vi "Calibration curve generator, inverse (for plot visualisation).vi"(0 "Calibration data":T1={"X cal.[]"=[0.18323830295620053, 0.5022759108677167, 0.5926494582411277, 0.6661572393359195, 0.7738522670991032, 0.8056162976693839, 0.8978854253288069, 0.9131465104685323, 0.998198602505461, 1.0026536354542668, 1.0697031684682123, 1.0921294784978217, 1.12634848007751], "Re cal.[]"=[0.05836901900647489, 0.22234941748039563, 0.3015014894413766, 0.37907259878050203, 0.5315212662031547, 0.5843186336351215, 0.7493379557739939, 0.7811312845686427, 0.9579100635301298, 0.968544779466997, 1.1278235480081842, 1.1845542549316277, 1.2707750850078616], "a1[]"=[0.5139845410306613, 0.694908421100499, 0.9655549133380104, 1.2354182702612118, 1.5388668488196042, 1.7253155968767342, 1.935875310920986, 2.080885331144939, 2.2328002605238204, 2.3813313947618693, 2.452594226248764, 2.5246632991683033], "a2[]"=[-0.567092642319511, 3.0111150428522957, -0.009461861177446703, 2.2004140825264833, 5.776179850523374, -0.22907956125341525, 19.477407826803766, -1.871103511573675, 70.58084557623488, -1.3220160025433672, 7.094218596447346, -0.2914365144530001], "a3[]"=[1.7775103256064757, -11.166529475918521, 16.733581628717324, -4.900141213800908, -59.63298736273686, 9.899216022714324, -643.3109334585097, 21.66651332028892, -8067.401298929666, 18.428518110921583, -163.1245085960374, 4.25840177969994]}, 5 "Overheat ratio":dbl=1.7, 7 "Gain":dbl=10.0, 9 "Offset (V)":dbl=0.512, 11 "N pts":i32=200, 12 "U_start (m/s)":dbl=0.3, 13 "U_end (m/s)":dbl=6.45, 14 "Ta (°C)":dbl=20.4383) -> ()   [LabVIEW 2022 SP3]
doc: "Generate spline interpolated calibration curve for plotting or testing purposes, inverse.\nPN 15-OCT-24."
uses:
  Ctls/Calibration data.ctl
  <vilib>/Analysis/1siggen.llb/Ramp Pattern by Samples.vi
  <vilib>/Analysis/NI_AALBase.lvlib
panel:
  out "U against Vout":cluster{dbl[], dbl[]}(graph)={[0.09565670008978011, 0.1343898964717316, 0.1737745519320799, 0.21373098990741246, 0.25415906989051273, 0.29493850771461716, 0.33593072128072055, 0.37698235326171226, 0.4179303781005761, 0.4586084143648783, 0.4988536102025265, 0.5385133294924527, 0.5774508898457986, 0.6155497865817461, 0.6527161209334209, 0.6888792508070907, 0.7239909224791807, 0.7580232803409792, 0.7909661871209617, 0.8228242441965239, 0.8536138157916306, 0.8833602633133519, 0.9120955076928228, 0.9398559684447683, 0.9666808802820959, 0.992610958957687, 1.017687373168673, 1.0419404638648222, 1.0648307784179123, 1.0863400234648268, 1.1067816169742883, 1.1263773140464783, 1.1452918887230468, 1.1636527433939259, 1.1815617818976187, 1.199103010231084, 1.216347641088802, 1.2333576762724352, 1.250188532885781, 1.2668910603604677, 1.2835131302849823, 1.3000737074622026, 1.3165183307523298, 1.3327837302632117, 1.3488125367586157, 1.3645549977294102, 1.3799700065077525, 1.3950254497808412, 1.409697968131386, 1.423972276022466, 1.4378402016851988, 1.4512995928993822, 1.4643532042626861, 1.4770174447515505, 1.489413910082965, 1.501590738566163, 1.5135643030588108, 1.5253492940795044, 1.5369589601284572, 1.5484053060396363, 1.5596992580108715, 1.5708508019310274, 1.5818691001255758, 1.592762590522131, 1.6035390713912545, 1.6142057741717097, 1.6247694263914259, 1.6352363063082798, 1.6456122905913884, 1.6559028961239342, 1.666113316817932, 1.6762484561786817, 1.6863129562336754, 1.6963112233410027, 1.706247451311157, 1.7161256422095328, 1.7259496251522843, 1.7357230733629458, 1.7454390277558163, 1.7549380938176284, 1.7642040931670222, 1.773280174660391, 1.782202692841075, 1.7910030846456615, 1.7997092295949835, 1.8083464784953251, 1.8169384687602363, 1.8255089240700306, 1.8340734713718665, 1.8426296175162848, 1.851173732752187, 1.8597022115890582, 1.8682114881290202, 1.8766980510068698, 1.8851584577645808, 1.893589348498953, 1.9019874586367636, 1.9103496307103862, 1.918672825027632, 1.9269541291519754, 1.9351907661324885, 1.943380101446166, 1.9515196486379371, 1.9596070736653148, 1.967640197974384, 1.9756170003516893, 1.9835356176118912, 1.9913943441939108, 1.9991916307484203, 2.00692608180709, 2.0145964526289784, 2.022201645322114, 2.029740704338787, 2.037212811441754, 2.044577031371202, 2.051621627394792, 2.0584422040883785, 2.0651575965089783, 2.071870086802438, 2.0786774895385776, 2.085550101994925, 2.092448142234443, 2.0993681711684484, 2.10630661311665, 2.1132597718178756, 2.1202238482677527, 2.127194960174401, 2.134169162776134, 2.141142470723861, 2.1481108806974722, 2.155070394401509, 2.162017041572377, 2.1689469026275665, 2.175856130597331, 2.18274097200035, 2.189597786355985, 2.1964230640655034, 2.2032134424409824, 2.2099657197115032, 2.216676866889371, 2.223344037432353, 2.229964574689168, 2.23653601716303, 2.243056101670474, 2.2495227645090354, 2.255934140776863, 2.2622885620099376, 2.2685845523181625, 2.274808698274382, 2.2806124757935544, 2.2863813895656646, 2.2922116126597114, 2.2980513875361175, 2.3038989912036323, 2.309752668696791, 2.3156106380566333, 2.32147109555613, 2.3273322211294523, 2.333192183960767, 2.3390491481853672, 2.344901278653928, 2.350746746709451, 2.3565837359260398, 2.3624104477592334, 2.3682251070589535, 2.374025967398322, 2.3798113161745906, 2.3855794794420593, 2.3913288264411303, 2.3970577737923513, 2.402764789329379, 2.408448395550149, 2.414107172670926, 2.4197397612733518, 2.4253448645398867, 2.430921250078122, 2.436466557075516, 2.44194958964132, 2.447368419589284, 2.45273726628724, 2.458069198680594, 2.463376486348948, 2.4686708978236394, 2.473963967621354, 2.479267249448951, 2.4845925713516106, 2.4899364329103912, 2.4952794764099337, 2.5006211554658653, 2.50596116144255, 2.511299185353878, 2.516634918044822, 2.521968050373835, 2.5272982733957337, 2.532625278544789, 2.537948757817723, 2.543268403956315, 2.5485839106292785, 2.5538949726131643, 2.559201285971937], [0.3, 0.3309045226130653, 0.36180904522613067, 0.392713567839196, 0.4236180904522613, 0.4545226130653266, 0.48542713567839196, 0.5163316582914572, 0.5472361809045226, 0.578140703517588, 0.6090452261306533, 0.6399497487437186, 0.670854271356784, 0.7017587939698493, 0.7326633165829146, 0.7635678391959799, 0.7944723618090452, 0.8253768844221105, 0.8562814070351759, 0.8871859296482412, 0.9180904522613065, 0.9489949748743718, 0.9798994974874371, 1.0108040201005026, 1.041708542713568, 1.0726130653266333, 1.1035175879396986, 1.1344221105527639, 1.1653266331658292, 1.1962311557788945, 1.2271356783919598, 1.2580402010050251, 1.2889447236180904, 1.319849246231156, 1.3507537688442213, 1.3816582914572866, 1.412562814070352, 1.4434673366834172, 1.4743718592964825, 1.5052763819095478, 1.5361809045226131, 1.5670854271356784, 1.5979899497487438, 1.628894472361809, 1.6597989949748744, 1.69070351758794, 1.7216080402010052, 1.7525125628140705, 1.7834170854271358, 1.8143216080402012, 1.8452261306532665, 1.8761306532663318, 1.907035175879397, 1.9379396984924624, 1.9688442211055277, 1.999748743718593, 2.030653266331658, 2.0615577889447234, 2.092462311557789, 2.1233668341708545, 2.15427135678392, 2.185175879396985, 2.2160804020100504, 2.2469849246231157, 2.277889447236181, 2.3087939698492463, 2.3396984924623117, 2.370603015075377, 2.4015075376884423, 2.4324120603015076, 2.463316582914573, 2.494221105527638, 2.5251256281407035, 2.556030150753769, 2.586934673366834, 2.6178391959798994, 2.6487437185929648, 2.67964824120603, 2.7105527638190954, 2.7414572864321607, 2.772361809045226, 2.8032663316582913, 2.8341708542713566, 2.865075376884422, 2.8959798994974872, 2.9268844221105526, 2.957788944723618, 2.988693467336683, 3.0195979899497485, 3.050502512562814, 3.0814070351758795, 3.112311557788945, 3.14321608040201, 3.1741206030150755, 3.205025125628141, 3.235929648241206, 3.2668341708542714, 3.2977386934673367, 3.328643216080402, 3.3595477386934673, 3.3904522613065327, 3.421356783919598, 3.4522613065326633, 3.4831658291457286, 3.514070351758794, 3.544974874371859, 3.5758793969849245, 3.60678391959799, 3.637688442211055, 3.6685929648241205, 3.6994974874371858, 3.730402010050251, 3.7613065326633164, 3.7922110552763817, 3.823115577889447, 3.8540201005025123, 3.884924623115578, 3.9158291457286434, 3.9467336683417087, 3.977638190954774, 4.00854271356784, 4.039447236180905, 4.07035175879397, 4.101256281407036, 4.132160804020101, 4.163065326633166, 4.193969849246232, 4.224874371859297, 4.255778894472362, 4.2866834170854275, 4.317587939698493, 4.348492462311558, 4.3793969849246235, 4.410301507537689, 4.441206030150754, 4.472110552763819, 4.503015075376885, 4.53391959798995, 4.564824120603015, 4.595728643216081, 4.626633165829146, 4.657537688442211, 4.688442211055277, 4.719346733668342, 4.750251256281407, 4.7811557788944725, 4.812060301507538, 4.842964824120603, 4.8738693467336685, 4.904773869346734, 4.935678391959799, 4.966582914572864, 4.99748743718593, 5.028391959798995, 5.05929648241206, 5.090201005025126, 5.121105527638191, 5.152010050251256, 5.182914572864322, 5.213819095477387, 5.244723618090452, 5.2756281407035175, 5.306532663316583, 5.337437185929648, 5.368341708542713, 5.399246231155779, 5.430150753768844, 5.461055276381909, 5.491959798994975, 5.52286432160804, 5.553768844221105, 5.584673366834171, 5.615577889447236, 5.646482412060301, 5.6773869346733665, 5.708291457286432, 5.739195979899497, 5.7701005025125625, 5.801005025125628, 5.831909547738693, 5.862814070351759, 5.893718592964825, 5.92462311557789, 5.955527638190955, 5.9864321608040205, 6.017336683417086, 6.048241206030151, 6.0791457286432165, 6.110050251256282, 6.140954773869347, 6.171859296482412, 6.202763819095478, 6.233668341708543, 6.264572864321608, 6.295477386934674, 6.326381909547739, 6.357286432160804, 6.38819095477387, 6.419095477386935, 6.45]}
  out "Calibration curve":cluster{dbl[], dbl[]}(graph)={[0.18451097716861914, 0.19652537347054594, 0.20883298963589056, 0.22141320587161856, 0.23423819544835056, 0.2472727548728119, 0.26047463068740484, 0.27379542336054125, 0.28718207192142786, 0.3005788254708218, 0.31392951339678693, 0.32717986335272775, 0.3402796056958915, 0.3531841487174906, 0.365855695129608, 0.3782637698457373, 0.3903852154178121, 0.40220376777841, 0.41370934729013237, 0.4248971946349325, 0.4357669584395782, 0.44632181214277844, 0.45656764901945185, 0.46651238062858197, 0.476165346624981, 0.48553683253197344, 0.4946376855652234, 0.5034751781541572, 0.5118480638703804, 0.5197440706361511, 0.5272735497260558, 0.5345146935617827, 0.5415257237079875, 0.5483517836440789, 0.5550291144751378, 0.5615877309369915, 0.5680532220324355, 0.574448018846105, 0.5807923288016678, 0.5871048588876737, 0.5934033913908016, 0.5996949027790756, 0.6059584418879481, 0.6121694791887384, 0.6183055074963921, 0.6243467367193586, 0.6302765339708374, 0.6360816054103551, 0.6417519511197015, 0.647280645556046, 0.6526635030850395, 0.6578986839495075, 0.6629862854029505, 0.667931779891953, 0.6727819095589543, 0.6775549708575999, 0.6822569237172977, 0.6868931198680651, 0.6914683899511406, 0.6959871154220011, 0.7004532883800795, 0.7048705617244951, 0.7092422914921751, 0.7135715728288287, 0.717861270736505, 0.722114046507269, 0.7263323805720736, 0.7305185923535991, 0.7346748576018877, 0.7388032236047495, 0.7429056225958743, 0.7469838836282733, 0.7510397431361439, 0.7550748543721464, 0.7590907958777113, 0.7630890791199043, 0.7670711554086191, 0.7710384221915293, 0.7749879608006575, 0.7788547416735615, 0.7826317994234272, 0.7863363737405534, 0.7899830259774788, 0.7935843855958696, 0.7971516922374349, 0.8006952069303505, 0.8042245394401007, 0.8077493836919192, 0.8112761457970955, 0.8148037882201684, 0.8183307989034609, 0.8218556684935193, 0.8253768967804789, 0.8288929990284882, 0.8324025121231073, 0.8359040004658274, 0.8393960615516053, 0.8428773311723734, 0.8463464881975853, 0.8498022588917484, 0.8532434207382498, 0.8566688057483318, 0.86007730324347, 0.8634678621085019, 0.8668394925212949, 0.8701912671724579, 0.8735223219953733, 0.8768318564325941, 0.8801191332693794, 0.8833834780687708, 0.8866242782452292, 0.8898409818154629, 0.8930330958657748, 0.8962001847751999, 0.8993247820360901, 0.9023167718094229, 0.9052164174744409, 0.9080740389004627, 0.9109330956825705, 0.9138353052238143, 0.9167681010577989, 0.9197145620290823, 0.922673248214591, 0.92564265566199, 0.9286212229289171, 0.9316073384512384, 0.9345993486571023, 0.937595566722432, 0.9405942818447109, 0.9435937688962538, 0.946592298306478, 0.9495881460155551, 0.9525796033395557, 0.9555649865899938, 0.9585426462983452, 0.9615109759082291, 0.9644684198139852, 0.9674134806434742, 0.9703447257042379, 0.9732607925346676, 0.9761603935246739, 0.9790423195925368, 0.9819054429254521, 0.9847487188100789, 0.987571186595719, 0.9903719698462261, 0.993150275747306, 0.995905393843459, 0.9986313815879183, 1.0011753287660317, 1.003705972126855, 1.0062655134444942, 1.0088312671174489, 1.011402485155225, 1.0139784031162342, 1.0165582422395538, 1.0191412116966452, 1.0217265109457183, 1.0243133321697613, 1.0269008627778182, 1.029488287948065, 1.0320747931904932, 1.0346595669066665, 1.0372418029240857, 1.0398207029831326, 1.0423954791553554, 1.0449653561730352, 1.0475295736514572, 1.050087388187049, 1.052638075316576, 1.0551809313247011, 1.057715274889572, 1.0602404485584174, 1.0627558200475489, 1.0652607833634884, 1.0677547597442336, 1.070236663710926, 1.072692487046901, 1.0751213044997503, 1.0775294344056343, 1.0799226971802045, 1.0823065708871378, 1.0846863238844942, 1.0870671340573013, 1.089454202411306, 1.0918528680992148, 1.0942615736420562, 1.0966716021014082, 1.099082705989238, 1.1014947445528838, 1.1039075764910384, 1.106321060035682, 1.1087350530347946, 1.1111494130356936, 1.1135639973688662, 1.1159786632321642, 1.1183932677752186, 1.1208076681839283, 1.1232217217648968, 1.1256352860296606], [0.059022239021742466, 0.06510241942347976, 0.07118259982521706, 0.07726278022695435, 0.08334296062869162, 0.08942314103042892, 0.09550332143216621, 0.10158350183390348, 0.1076636822356408, 0.11374386263737808, 0.11982404303911538, 0.12590422344085264, 0.13198440384258997, 0.13806458424432724, 0.14414476464606454, 0.15022494504780184, 0.15630512544953912, 0.1623853058512764, 0.1684654862530137, 0.174545666654751, 0.18062584705648826, 0.18670602745822554, 0.19278620785996284, 0.19886638826170014, 0.20494656866343747, 0.21102674906517474, 0.217106929466912, 0.2231871098686493, 0.2292672902703866, 0.23534747067212386, 0.2414276510738612, 0.24750783147559846, 0.2535880118773357, 0.25966819227907306, 0.26574837268081036, 0.27182855308254766, 0.2779087334842849, 0.2839889138860222, 0.2900690942877595, 0.2961492746894968, 0.30222945509123406, 0.30830963549297136, 0.3143898158947086, 0.32046999629644596, 0.32655017669818326, 0.33263035709992056, 0.33871053750165786, 0.3447907179033951, 0.3508708983051324, 0.3569510787068697, 0.36303125910860695, 0.36911143951034425, 0.3751916199120816, 0.3812718003138188, 0.38735198071555615, 0.39343216111729346, 0.3995123415190307, 0.40559252192076795, 0.4116727023225053, 0.4177528827242426, 0.4238330631259799, 0.42991324352771715, 0.43599342392945445, 0.4420736043311918, 0.44815378473292905, 0.45423396513466635, 0.46031414553640365, 0.4663943259381409, 0.4724745063398782, 0.4785546867416155, 0.48463486714335274, 0.49071504754509004, 0.49679522794682734, 0.5028754083485646, 0.5089555887503019, 0.5150357691520392, 0.5211159495537765, 0.5271961299555138, 0.5332763103572511, 0.5393564907589883, 0.5454366711607257, 0.551516851562463, 0.5575970319642002, 0.5636772123659375, 0.5697573927676748, 0.5758375731694121, 0.5819177535711494, 0.5879979339728867, 0.5940781143746239, 0.6001582947763612, 0.6062384751780985, 0.6123186555798359, 0.6183988359815732, 0.6244790163833105, 0.6305591967850478, 0.6366393771867851, 0.6427195575885223, 0.6487997379902596, 0.6548799183919969, 0.6609600987937342, 0.6670402791954715, 0.6731204595972088, 0.679200639998946, 0.6852808204006833, 0.6913610008024206, 0.6974411812041579, 0.7035213616058952, 0.7096015420076325, 0.7156817224093697, 0.721761902811107, 0.7278420832128443, 0.7339222636145816, 0.740002444016319, 0.7460826244180563, 0.7521628048197935, 0.7582429852215308, 0.7643231656232682, 0.7704033460250055, 0.7764835264267427, 0.78256370682848, 0.7886438872302174, 0.7947240676319547, 0.8008042480336919, 0.8068844284354292, 0.8129646088371665, 0.8190447892389038, 0.8251249696406411, 0.8312051500423785, 0.8372853304441156, 0.8433655108458529, 0.8494456912475903, 0.8555258716493276, 0.8616060520510649, 0.8676862324528022, 0.8737664128545394, 0.8798465932562767, 0.885926773658014, 0.8920069540597513, 0.8980871344614886, 0.9041673148632258, 0.9102474952649631, 0.9163276756667004, 0.9224078560684377, 0.928488036470175, 0.9345682168719123, 0.9406483972736495, 0.9467285776753868, 0.9528087580771241, 0.9588889384788614, 0.9649691188805987, 0.971049299282336, 0.9771294796840732, 0.9832096600858105, 0.9892898404875479, 0.9953700208892852, 1.0014502012910225, 1.0075303816927597, 1.0136105620944968, 1.0196907424962343, 1.0257709228979714, 1.0318511032997089, 1.037931283701446, 1.0440114641031835, 1.0500916445049207, 1.0561718249066578, 1.0622520053083953, 1.0683321857101327, 1.0744123661118699, 1.0804925465136073, 1.0865727269153445, 1.0926529073170816, 1.098733087718819, 1.1048132681205562, 1.1108934485222937, 1.1169736289240308, 1.123053809325768, 1.1291339897275054, 1.1352141701292426, 1.14129435053098, 1.1473745309327172, 1.1534547113344549, 1.159534891736192, 1.1656150721379295, 1.1716952525396667, 1.1777754329414039, 1.1838556133431413, 1.1899357937448785, 1.1960159741466159, 1.202096154548353, 1.2081763349500905, 1.2142565153518277, 1.220336695753565, 1.2264168761553023, 1.2324970565570394, 1.2385772369587769, 1.244657417360514, 1.2507375977622515, 1.2568177781639887, 1.2628979585657258, 1.2689781389674633]}
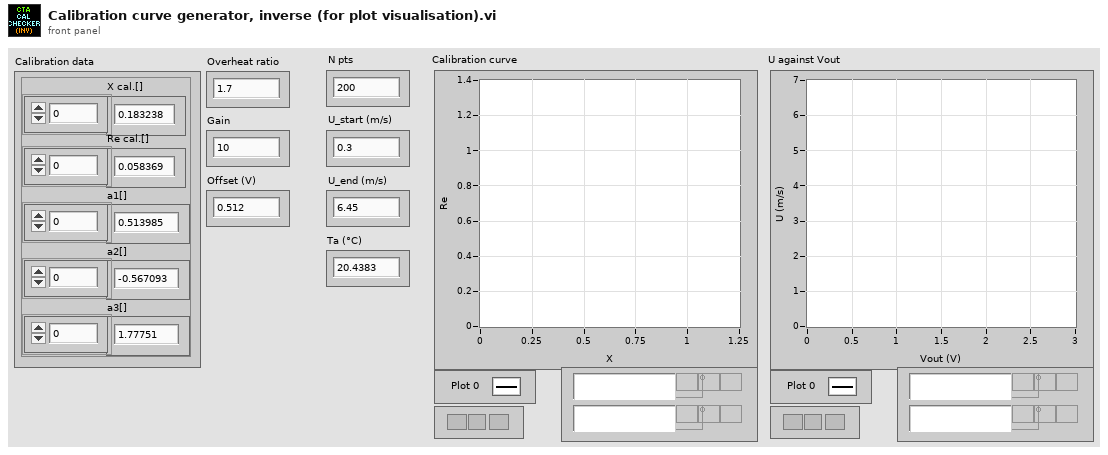
[diagram p1: front panel]
types:
  T1 = typedef "Calibration data.ctl" = cluster{"X cal.[]":dbl[], "Re cal.[]":dbl[], "a1[]":dbl[], "a2[]":dbl[], "a3[]":dbl[]}
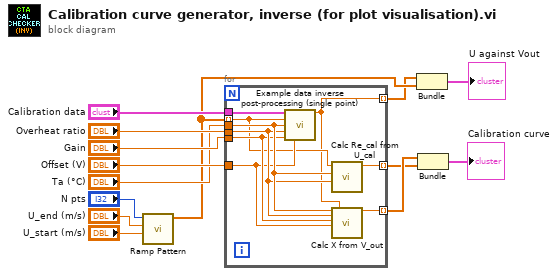
[diagram p0: block diagram]
diagram:
  n1 = call-poly <vilib>:"Ramp Pattern.vi"("start"="U_start (m/s)", "end"="U_end (m/s)", "samples"="N pts") -> ("Ramp Pattern"=w2:dbl[])  [unwired: 7 in, 1 out]
  n2 = for {
    tunnel: "Offset (V)" -> [w17]
    tunnel: "Gain" -> [w18]
    tunnel: "Overheat ratio" -> [w19]
    tunnel: "Calibration data" -> [w23]
    tunnel: w2 -> [w16] mode=indexing
    tunnel: "Ta (°C)" -> [w20]
    tunnel: [w22] -> w5 mode=indexing
    tunnel: [w21] -> w6 mode=indexing
    tunnel: [w15] -> w1 mode=indexing
    n3 = call "Example data inverse post-processing (single point).vi"("Calibration data"=w23, "U (m/s)"=w16, "Ta (°C)"=w20, "Overheat ratio (Rw / R0)"=w19, "Gain"=w18, "Offset (V)"=w17) -> ("V_out (V)"=w15:dbl)  [unwired: 9 in]
    n4 = call "Calc Re_cal from U_cal.vi"("Overheat ratio (Rw / R0)"=w19, "Ta (°C)"=w20, "U_cal (m/s)"=w16) -> ("Re"=w22:dbl)  [unwired: 8 in]
    n5 = call "Calc X from V_out.vi"("Ta (°C)"=w20, "Overheat ratio (Rw / R0)"=w19, "Gain"=w18, "Offset (V)"=w17, "V_out (V)"=w15) -> ("X"=w21:dbl)  [unwired: 14 in]
  }
  n6 = Bundle(w1, "Ramp Pattern"=w2) -> (→"U against Vout":cluster{dbl[], "Ramp Pattern":dbl[]})  [unwired: 1 in]
  n7 = Bundle(w6, w5) -> (→"Calibration curve":cluster{dbl[], dbl[]})  [unwired: 1 in]
